vi "tag array to filter table.vi"(8 "error in":errorcluster, 10 "filter":string, 11 "tag list":refnum<class "tag descriptor.lvclass">[](array[class])) -> (0 "error out":errorcluster, 3 "filter table":string[][](array[string]))   [LabVIEW 2013, in "PL Framework Configuration Tool.lvlib" / "EngineTags.lvclass"]
uses:
  EngineTags.lvclass
  <vilib>/NI/Tag Bus/tag/tag descriptor.lvclass
  <vilib>/NI/Tag Bus/tag/tag descriptor.lvclass/tag descriptor.ctl
  <vilib>/NI/Tag Bus/tag/read tag name.vi
  <vilib>/NI/Tag Bus/tag/read data type.vi
  <vilib>/NI/Tag Bus/tag/read metadata.vi
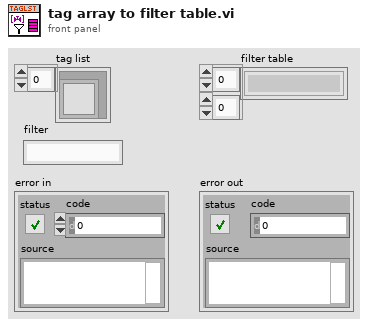
[diagram p1: front panel]
types:
  T1 = typedef "tag bus.lvlib/tag descriptor.lvclass/Data Type.ctl" = enum16{"Double", "Single", "I64", "I32", "I16", "I8", "U64", "U32", "U16", "U8", "Boolean", "String", "Array of Double", "Array of Single", "Array of I64", "Array of I32", "Array of I16", "Array of I8", "Array of U64", "Array of U32", "Array of U16", "Array of U8", "Array of Boolean", "Array of String"}
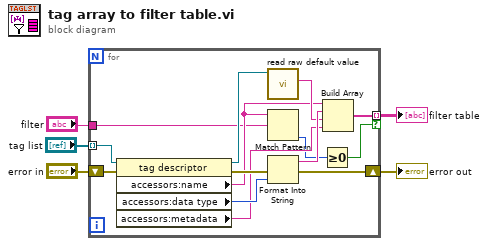
[diagram p0: block diagram]
diagram:
  n1 = for {
    shift-right: [w16] -> w5
    shift-left: "error in" -> [w19]
    tunnel: "tag list" -> [w18] mode=indexing
    tunnel: [w10] -> w2 mode=indexing if=w6
    tunnel: "filter" -> [w8]
    n2 = property class="tag descriptor"(reference=w18, error in=w19) -> (reference out=w14:refnum<class "tag descriptor.lvclass">, error out=w17:errorcluster, "accessors:name"=w9:string, "accessors:data type"=w15:T1, "accessors:metadata"=w12:string)
    n3 = call <vilib>:"read raw default value.vi"("system tag in"=w14) -> ("raw default"=w11:string)  [unwired: 8 in, 2 out]
    n4 = Match Pattern(string=w9, regular expression=w8) -> (offset past match=w7:i32)  [unwired: 1 in, 3 out]
    n5 = Format Into String(error in=w17, w15) -> (resulting string=w13:string, error out=w16:errorcluster)  [unwired: 2 in]
    n6 = Greater Or Equal To 0?(x=w7) -> (x >= 0?=w6:bool)
    n7 = Build Array(w9, w13, w11, w12) -> (w10:string[])
  }
  "error out" <- w5
  "filter table" <- w2
